vi "getUserEvents.vi"(11 "Publisher in":refnum<class "Publisher.lvclass">) -> (2 "UserEvents":refnum<class "UserEvents.lvclass">, 3 "Publisher out":refnum<class "Publisher.lvclass">)   [LabVIEW 2016, in "Publisher.lvclass"]
uses:
  Publisher.lvclass
  UserEvents/UserEvents.lvclass
  Publisher.lvclass/Publisher.ctl
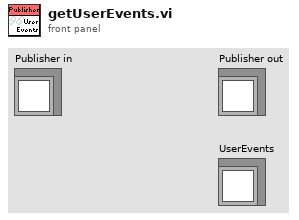
[diagram p1: front panel]
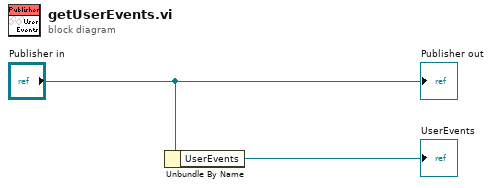
[diagram p0: block diagram]
diagram:
  n1 = Unbundle By Name("Publisher in") -> ("UserEvents"=→"UserEvents":refnum<class "UserEvents.lvclass">)
  "Publisher out" <- "Publisher in"
